vi "Configure Pulse Mode.vi"(7 "Enable Pulse Mode (T: Enable)":bool=TRUE, 8 "error in (no error)":errorcluster, 9 "Pulse Delay (.001 s)":dbl=0.001, 10 "Pulse Width (.0001 s)":dbl=0.0001, 11 "VISA resource name":refnum<visa-resource-name>) -> (0 "error out":errorcluster, 3 "VISA resource name out":refnum<visa-resource-name>)   [LabVIEW 2015, in "Keithley 24XX.lvlib"]
doc: "Enables and configures pulse mode settings on the instrument.\n\n<B>Note:</B> Pulse mode is only found on the 2430 mode. Also, pulse mode is incompatible with many of the other commands found on the instrument."
uses:
  <instrlib>/Keithley 24XX/Keithley 24XX.lvlib
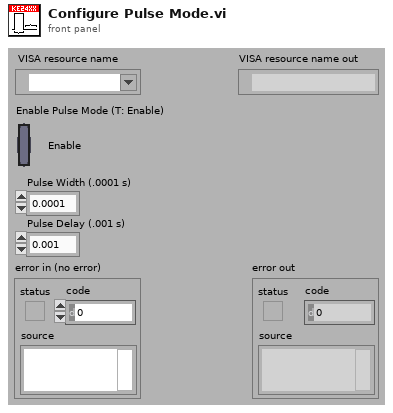
[diagram p1: front panel]
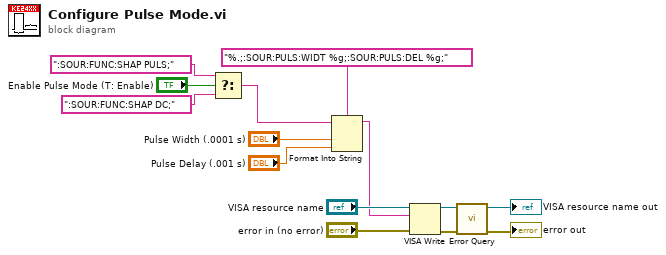
[diagram p0: block diagram]
diagram:
  n1 = Select(t=":SOUR:FUNC:SHAP PULS;", s="Enable Pulse Mode (T: Enable)", f=":SOUR:FUNC:SHAP DC;") -> (s? t:f=w4:string)
  n2 = Format Into String(format string="%.;:SOUR:PULS:WIDT %g;:SOUR:PULS:DEL %g;", initial string=w4, "Pulse Width (.0001 s)", "Pulse Delay (.001 s)") -> (resulting string=w3:string)  [unwired: 1 in, 1 out]
  n3 = VISA Write(VISA resource name="VISA resource name", write buffer=w3, error in (no error)="error in (no error)") -> (VISA resource name out=w11:refnum<visa-resource-name>, error out=w10:errorcluster)  [unwired: 1 out]
  n4 = call <instrlib>:"Error Query.vi"("error in (no error)"=w10, "VISA resource name"=w11) -> ("error out"=→"error out":errorcluster, "VISA resource name out"=→"VISA resource name out":refnum<visa-resource-name>)  [unwired: 6 in, 2 out]
